vi "Create Statement from SQL.vi"(8 "error in (no error)":errorcluster, 9 "Num records":i32, 10 "SQL Dataset":variant[][](array[variant]), 11 "First Importing Transaction":refnum<class "Banking Record.lvclass">) -> (0 "error out":errorcluster, 3 "Overlapping Records":refnum<class "Statement.lvclass">)   [LabVIEW 2018, in "Banking Record.lvclass"]
uses:
  Banking Record.lvclass
  C:/Users/jtipps/Documents/Filthy-Lucre-Budgetizer/source/support/classes/Transaction/Transaction.lvclass
  Statement/Statement.lvclass
  Banking Statement/Banking Statement.lvclass
  C:/Users/jtipps/Documents/Filthy-Lucre-Budgetizer/source/support/classes/Statement/Statement.lvclass
  <vilib>/Utility/error.llb/DialogType.ctl
  Statement/Statement.lvclass/Statement.ctl
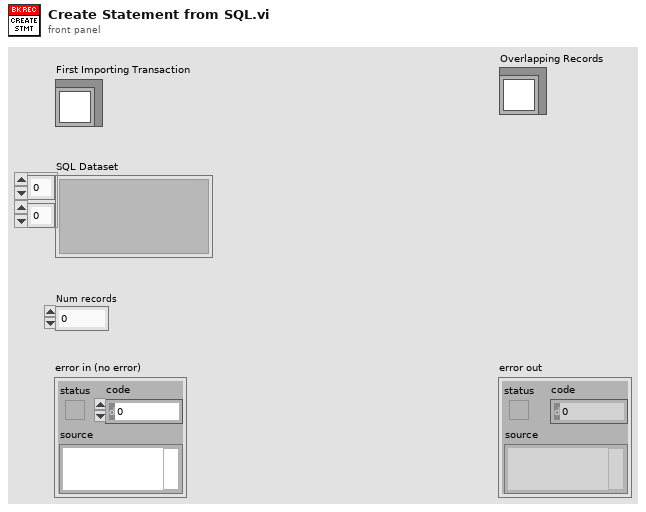
[diagram p1: front panel]
types:
  T1 = typedef "DialogType.ctl" = u16
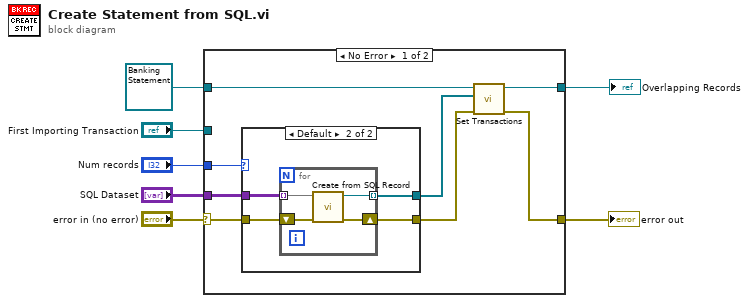
[diagram p0: block diagram]
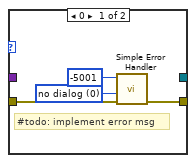
[diagram p2: hidden frame]
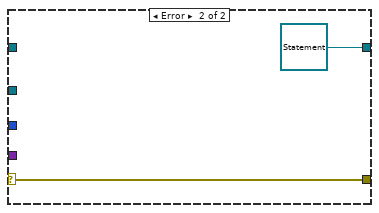
[diagram p3: hidden frame]
diagram:
  n1 = case shown="No Error" "error in (no error)" {
    selector: "error in (no error)" -> [w15 w29]
    tunnel: "Num records" -> [w14 _]
    tunnel: refnum<class "Banking Statement.lvclass"> refnum ("Banking Statement.lvclass") -> [w12 _]
    tunnel: "SQL Dataset" -> [w13 _]
    tunnel: "First Importing Transaction" -> [_ _]
    tunnel: [w8 w29] -> w3
    tunnel: [w11 refnum<class "Statement.lvclass"> refnum ("Statement out")] -> w1
    frame No Error {
      n2 = case shown="Default" w14 {
        tunnel: w15 -> [w18 w23]
        tunnel: [w19 w22] -> w9
        tunnel: w13 -> [_ w21]
        tunnel: [_ w20] -> w10
        frame 0 {
          w16 = T1 0 items=["no dialog", "OK message", "continue or stop message", "OK message + warnings", "continue/stop + warnings"] ("type of dialog (OK msg:1)")
          # "#todo: implement error msg"
          n3 = call <vilib>:"Simple Error Handler.vi"("error code (no error:0)"=-5001, "type of dialog (OK msg:1)"=w16, "error in (no error)"=w18) -> ("error out"=w19:errorcluster)  [unwired: 2 in, 4 out]
        }
        frame Default {
          n4 = for {
            shift-right: [w26] -> w22
            shift-left: w23 -> [w27]
            tunnel: w21 -> [w25] mode=indexing
            tunnel: [w24] -> w20 mode=indexing
            n5 = call "Create from SQL Record.vi"("error in (no error)"=w27, "MySQL Record"=w25) -> ("error out"=w26:errorcluster, "Banking Record"=w24:refnum<class "Banking Record.lvclass">)  [unwired: 8 in]
          }
        }
      }
      n6 = call "Set Transactions.vi"("error in (no error)"=w9, "Transactions"=w10, "Statement in"=w12) -> ("error out"=w8:errorcluster, "Statement out"=w11:refnum<class "Banking Statement.lvclass">)  [unwired: 7 in]
    }
    frame Error {
    }
  }
  "error out" <- w3
  "Overlapping Records" <- w1
